vi "Test Set Motor Velocity.vi"() -> ()   [LabVIEW 2017]
uses:
  <vilib>/Platform/TimedLoop/XDataNode/timing_clust.ctl
  <vilib>/Platform/TimedLoop/XDataNode/nitl_modes.ctl
  <vilib>/Platform/TimedLoop/XDataNode/wakeup.ctl
  <vilib>/Platform/TimedLoop/XDataNode/XDataNode.xnode
  <vilib>/Platform/TimedLoop/XDataNode/XDNodeRunTimeDep.lvlib
panel:
  in  "Left motor speed rev/s":dbl
  in  "Right motor speed rev/s":dbl
  in  "Disable motors":bool
  in  "Accelerate?":bool=TRUE
  in  "Acceleration ramp constant":dbl(slide)=10.303030303030303 scale=0.0..20.0
  in  "stop":bool
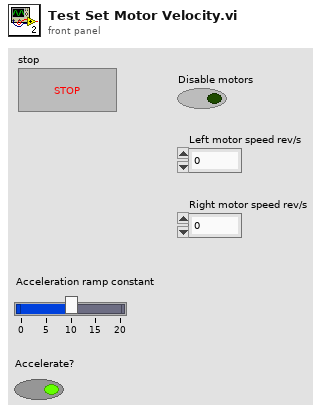
[diagram p1: front panel]
types:
  T1 = typedef "XDNodeRunTimeDep.lvlib/timing_clust.ctl" = cluster{"Expected End [f-1]":u64, "Actual End [f-1]":u64, "Finished Late? [f-1]":bool, "Expected End [i-1]":u64, "Actual End [i-1]":u64, "Finished Late? [i-1]":bool, "Expected Start [i]":u64, "Actual Start [i]":u64, "Expected Start [f]":u64, "Actual Start [f]":u64, "Source Name":string, "Structure Name":string, "Period":i64, "Deadline":i64, "Offset":i64, "Start":i64, "Priority":i32, "Timeout":i32, "Mode":T2, "Wakeup Reason":T3, "Error":errorcluster, "Source Type":string, "Secondary Source Type":string, "Global End Time":u64, "Global Start Time":u64, "Frame Duration":u64, "Iteration Duration":u64, "Assigned CPU":i32, "I/O Scan Engine Mode":u32}
  T2 = typedef "XDNodeRunTimeDep.lvlib/nitl_modes.ctl" = enum32{"No Change", "Process missed periods, maintain original phase", "Discard missed periods, maintain original phase", "Process missed periods, ignore original phase", "Discard missed periods, ignore original phase"}
  T3 = typedef "XDNodeRunTimeDep.lvlib/wakeup.ctl" = enum32{"Normal", "Aborted", "Asynchronous wakeup", "Timing source error", "Timed loop error", "Timeout"}
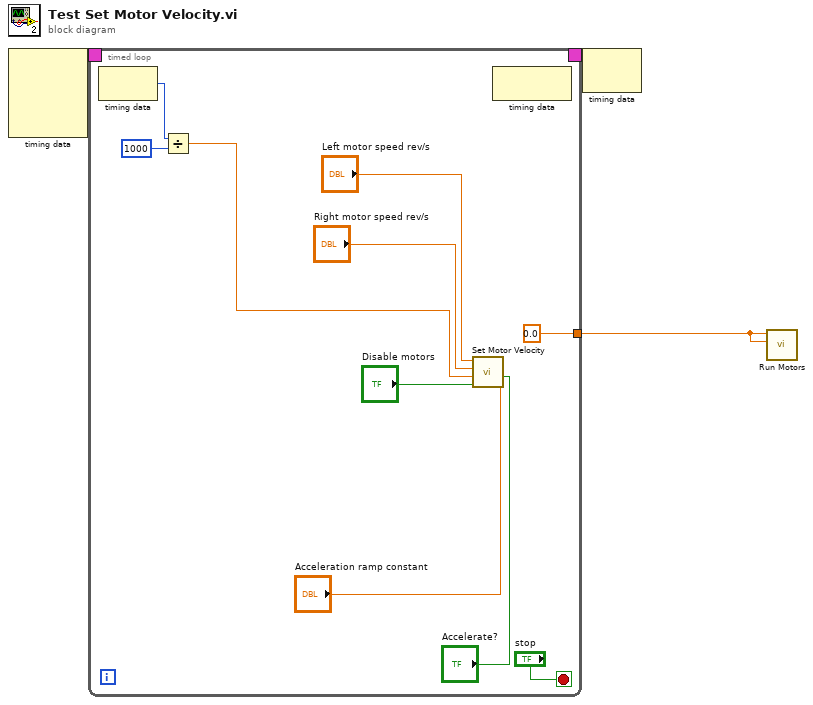
[diagram p0: block diagram]
diagram:
  n1 = node-c288() -> (w3:T1)  [unwired: 4 in]
  n2 = timed-loop {
    timing: w3 -> [_]
    timing-out: [_] -> w2
    tunnel: [0.0 ("Right motor side (-1..1)")] -> w1
    stop <- "stop" stop-if-true
    n3 = node-c288() -> (w7:i64)  [unwired: 1 in]
    n4 = Divide(x=w7, y=i64 1000) -> (x/y=w5:dbl)
    n5 = call "Set Motor Velocity.vi"("Acceleration ramp constant"="Acceleration ramp constant", "Accelerate?"="Accelerate?", "Disable motors"="Disable motors", "dt"=w5, "Right motor speed rev/s"="Right motor speed rev/s", "Left motor speed rev/s"="Left motor speed rev/s") -> ()  [unwired: 6 in]
    n6 = node-c288() -> ()  [unwired: 1 in, 1 out]
  }
  n7 = node-c288(w2) -> ()  [unwired: 1 out]
  n8 = call "Run Motors.vi"("Right motor side (-1..1)"=w1, "Left motor speed (-1..1)"=w1) -> ()  [unwired: 10 in]
